vi "Win Host - Update Formatting.vi"(8 "error in (no error)":errorcluster, 9 "Short-Cut?":bool, 10 "Index":i32, 11 "Control in":refnum<vi>) -> (0 "error out":errorcluster)   [LabVIEW 2024]
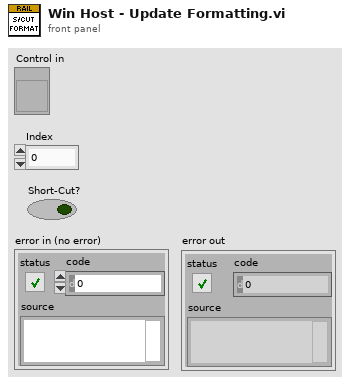
[diagram p1: front panel]
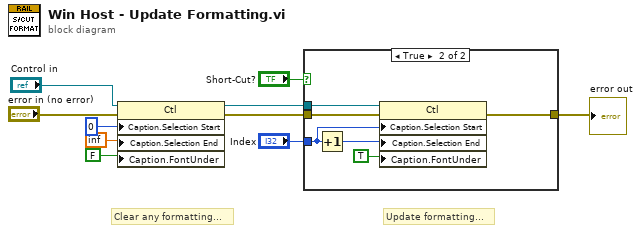
[diagram p0: block diagram]
diagram:
  # "Update formatting..."
  # "Clear any formatting..."
  n1 = property class="Ctl"(reference="Control in", error in="error in (no error)", "Caption.Selection Start"=u32 0 ("Text.Selection:Start"), "Caption.Selection End"=inf, "Caption.FontUnder"=FALSE) -> (reference out=w1:refnum<vi>, error out=w10:errorcluster)
  n2 = case shown="True" "Short-Cut?" {
    tunnel: "Index" -> [_ w17]
    tunnel: w10 -> [w11 w14]
    tunnel: [w11 w13] -> w2
    tunnel: w1 -> [_ w12]
    frame False {
    }
    frame True {
      n3 = Increment(x=w17) -> (x+1=w16:i32)
      n4 = property class="Ctl"(reference=w12, error in=w14, "Caption.Selection Start"=w17, "Caption.Selection End"=w16, "Caption.FontUnder"=TRUE ("Caption.Font:Underline")) -> (error out=w13:errorcluster)  [unwired: 1 out]
    }
  }
  "error out" <- w2
